vi "Trace_Enable.vi"(6 "Calltree level":i32, 9 "Category":string) -> (1 "TraceEnabled":bool)   [LabVIEW 2018]
uses:
  protected/Tracer_ClassAttributes.vi
  Tracer.lvclass
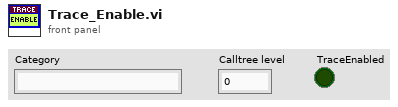
[diagram p1: front panel]
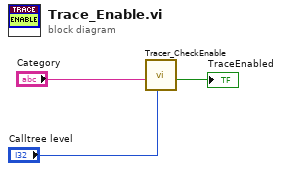
[diagram p0: block diagram]
diagram:
  n1 = call "Tracer_CheckEnable.vi"("Calltree level"="Calltree level", "Category"="Category") -> ("TraceEnabled"=→"TraceEnabled":bool)  [unwired: 9 in]
